vi "MainPresentor2.vi"() -> ()   [LabVIEW 2010]
uses:
  <vilib>/Utility/miscctls.llb/LV3DPointTypeDef.ctl
  <vilib>/Utility/miscctls.llb/LVPositionTypeDef.ctl
  LVPresent_Globals.vi
panel:
  in  "Done":bool
  out "#":i16
  out "ScanCode":i16
  out "3D Picture":refnum<vi>(3d-picture)
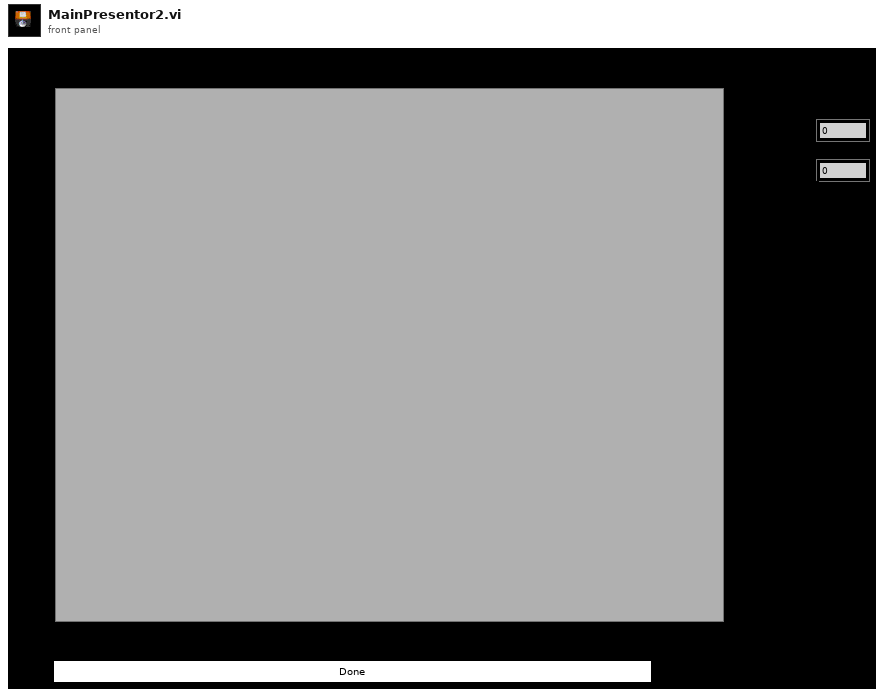
[diagram p1: front panel]
types:
  T1 = typedef "LV3DPointTypeDef.ctl" = cluster{"X":sgl, "Y":sgl, "Z":sgl}
  T2 = typedef "LVPositionTypeDef.ctl" = cluster{"Left":i32, "Top":i32}
  T3 = typedef "LVBoundsTypeDef.ctl" = cluster{"Width":u32, "Height":u32}
  T4 = typedef "LVRectTypeDef.ctl" = cluster{"left":i16, "top":i16, "right":i16, "bottom":i16}
  T5 = typedef "SlideTypeDef.ctl" = cluster{"Slide path":string, "Transition":enum16{"Pan", "Zoom-pan-zoom", "Zoom-wait-Zoom"}, "frame":cluster{"left":i16, "top":i16, "right":i16, "bottom":i16}, "Number":i32}
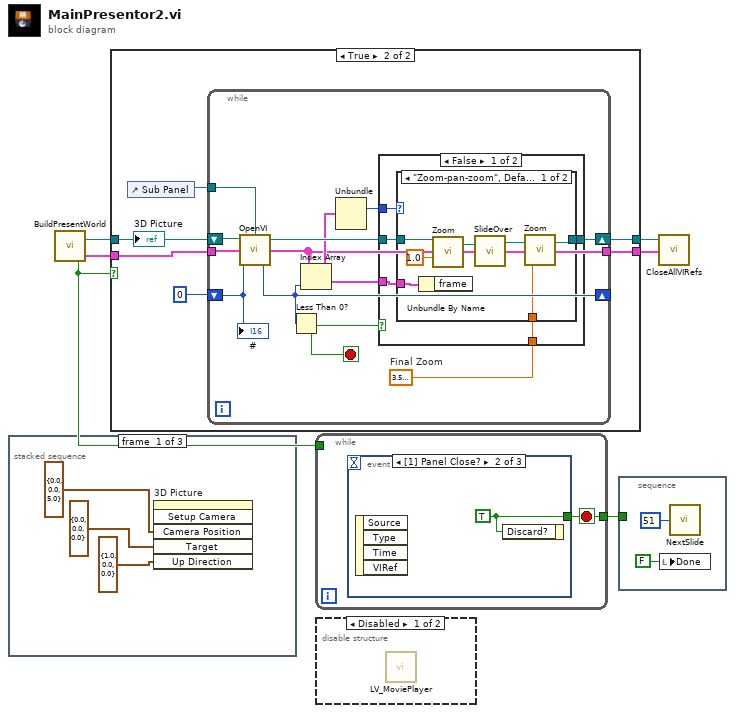
[diagram p0: block diagram]
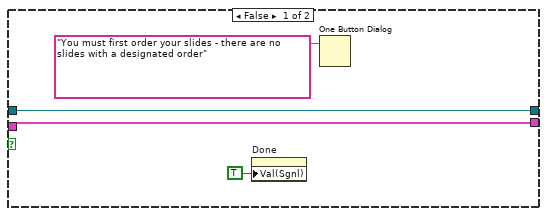
[diagram p2: hidden frame]
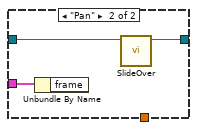
[diagram p3: hidden frame]
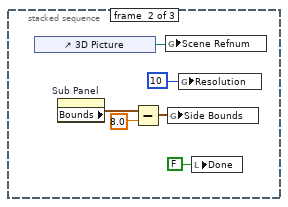
[diagram p6: hidden frame]
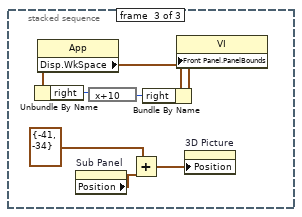
[diagram p7: hidden frame]
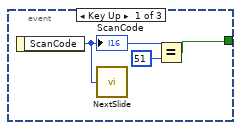
[diagram p8: hidden frame]
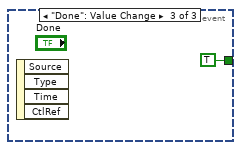
[diagram p9: hidden frame]
diagram:
  n1 = stacked-sequence {
    frame #0 {
      n2 = invoke on="3D Picture" class="SceneGraphDisp (strict)" method="Setup Camera"("Camera Position"=T1 {"X"=0.0, "Y"=0.0, "Z"=5.0}, "Target"=T1 {"X"=0.0, "Y"=0.0, "Z"=0.0}, "Up Direction"=T1 {"X"=1.0, "Y"=0.0, "Z"=0.0}) -> ()  [unwired: 3 in, 6 out]
    }
    frame #1 {
      n3 = control-ref of="3D Picture"() -> (w11:refnum<vi>)
      n4 = property on="Sub Panel" class="SubPnl"() -> ("Bounds"=w13:T3)  [unwired: 2 in, 2 out]
      n5 = Subtract(x=w13, y=8.0) -> (x-y=w14:cluster{"Width":dbl, "Height":dbl})
      n6 = global write "LVPresent_Globals.vi" "Scene Refnum"(w11) -> ()
      n7 = global write "LVPresent_Globals.vi" "Side Bounds"(w14) -> ()
      n8 = global write "LVPresent_Globals.vi" "Resolution"(10 ("Resolution")) -> ()
      n9 = local write "Done"(FALSE ("Done")) -> ()
    }
    frame #2 {
      n10 = property class="App"() -> ("Disp.WkSpace"=w18:T4)  [unwired: 2 in, 2 out]
      n11 = Unbundle By Name(w18) -> ("right"=w16:i16)
      n12 = property on="Sub Panel" class="SubPnl"() -> ("Position"=w20:T2)  [unwired: 2 in, 2 out]
      n13 = expression code="x+10"(w16) -> (w17:i16)
      n14 = Add(x=T2 {"Left"=-41, "Top"=-34} ("x-y"), y=w20) -> (x+y=w22:T2)
      n15 = Bundle By Name(cluster=w18, "right"=w17) -> (w19:T4)
      n16 = property class="VI"("Front Panel.PanelBounds"=w19) -> ()  [unwired: 2 in, 2 out]
      n17 = property on="3D Picture" class="SceneGraphDisp (strict)"("Position"=w22) -> ()  [unwired: 2 in, 2 out]
    }
  }
  n18 = call "BuildPresentWorld.vi"() -> ("Valid slides?"=w1:bool, "SlideInfo"=w4:T5[], "Scene.Object Out"=w5:refnum<vi>)  [unwired: 2 in]
  n19 = case shown="True" w1 {
    tunnel: w5 -> [w26 w31]
    tunnel: w4 -> [w25 w29]
    tunnel: [w26 w28] -> w3
    tunnel: [w25 w27] -> w2
    frame False {
      n20 = property on="Done" class="Bool (strict)"("Val(Sgnl)"=TRUE ("Value (Signaling)")) -> ()  [unwired: 2 in, 2 out]
      n21 = One Button Dialog(message="You must first order your slides - there are no slides with a designated order") -> ()  [unwired: 1 in, 1 out]
    }
    frame True {
      n22 = control-ref of="Sub Panel"() -> (w30:refnum<vi>)
      n23 = while {
        shift-right: [w43] -> w28
        shift-left: w31 -> [w42]
        tunnel: w30 -> [w41]
        shift-right: [w37] -> _
        shift-left: 0 ("Resolution") -> [w34]
        tunnel: w29 -> [w38]
        tunnel: [w38] -> w27
        stop <- w33 stop-if-true
        w36 = sgl 3.6  # Final Zoom
        n24 = call "OpenVI.vi"("#"=w34, "Slides"=w38, "Scene.Object in"=w42, "reference"=w41) -> ("New #"=w37:i32, "Scene.Object Out"=w40:refnum<vi>)
        n25 = Less Than 0?(x=w37) -> (x < 0?=w33:bool)
        n26 = Index Array(array=w38, index=w37) -> (element=w39:T5)
        n27 = Unbundle(w39) -> ("Transition"=w35:enum16{"Pan", "Zoom-pan-zoom", "Zoom-wait-Zoom"})  [unwired: 3 out]
        n28 = case shown="False" w33 {
          tunnel: [w46 w59] -> w43
          tunnel: w40 -> [w47 w59]
          tunnel: w39 -> [w48 _]
          tunnel: w35 -> [w45 _]
          tunnel: w36 -> [w44 _]
          frame False {
            n29 = case shown="\"Zoom-pan-zoom\", Default" w45 {
              tunnel: w48 -> [w51 w56]
              tunnel: w47 -> [w54 w57]
              tunnel: [w52 w58] -> w46
              tunnel: w44 -> [w49 _]
              frame "Zoom-pan-zoom", Default {
                n30 = Unbundle By Name(w51) -> ()  [unwired: 1 out]
                n31 = call "Zoom.vi"("Final Zoom"=sgl 1.0, "Scene.Object IN"=w54) -> ("Scene.Object Out"=w53:refnum<vi>)  [unwired: 1 in]
                n32 = call "SlideOver.vi"("Scene.Object IN"=w53) -> ("Scene.Object Out"=w50:refnum<vi>)  [unwired: 2 in]
                n33 = call "Zoom.vi"("Final Zoom"=w49, "Scene.Object IN"=w50) -> ("Scene.Object Out"=w52:refnum<vi>)  [unwired: 1 in]
              }
              frame "Pan" {
                n34 = Unbundle By Name(w56) -> ()  [unwired: 1 out]
                n35 = call "SlideOver.vi"("Scene.Object IN"=w57) -> ("Scene.Object Out"=w58:refnum<vi>)  [unwired: 2 in]
              }
            }
          }
          frame True {
          }
        }
        "#" <- w34
      }
      "3D Picture" <- w31
    }
  }
  n36 = while {
    tunnel: [w60] -> w6
    tunnel: w1 -> [_]
    stop <- w60 stop-if-true
    n37 = event shown="[1] Panel Close?" {
      selector: _ -> [_ _ _]
      dyn-events: _ -> [_ _ _]
      timeout: _ -> [_ _ _]
      tunnel: [w62 w64 TRUE] -> w60
      event Key Up {
        n38 = event-data() -> ("ScanCode"=w63:i16)  [unwired: 1 in]
        "ScanCode" <- w63
        n39 = call "NextSlide.vi"("ScanCode"=w63) -> ()  [unwired: 1 out]
        n40 = Equal?(x=w63, y=i16 51 ("ScanCode")) -> (x = y?=w62:bool)
      }
      event Panel Close? {
        w64 = TRUE
        n41 = event-data() -> ()  [unwired: 1 in, 4 out]
        n42 = event-data("Discard?"=w64) -> ()  [unwired: 1 in, 1 out]
      }
      event "Done": Value Change {
        n43 = event-data() -> ()  [unwired: 1 in, 4 out]
      }
    }
  }
  n44 = disable-structure shown="Disabled" {
    frame Disabled {
      n45 = call "LV_MoviePlayer.vi"() -> ()  [unwired: 5 in, 1 out]
    }
    frame Enabled {
    }
  }
  n46 = stacked-sequence {
    tunnel: w6 -> [_]
    frame #0 {
      n47 = local write "Done"(FALSE ("Done")) -> ()
      n48 = call "NextSlide.vi"("ScanCode"=i16 51) -> ()  [unwired: 1 out]
    }
  }
  n49 = call "CloseAllVIRefs.vi"("SlideInfo"=w2, "Scene.Object IN"=w3) -> ()  [unwired: 1 in]
